vi "Image Processing Module Event Handler.vi"(8 "error in (no error)":errorcluster, 9 "data queue":refnum<queue>, 10 "Data Event":refnum<user-event>) -> ()   [LabVIEW 2018, in "Headless Image Processing Handler.lvclass"]
uses:
  Headless Image Processing Handler.lvclass
  Message/Message.lvclass
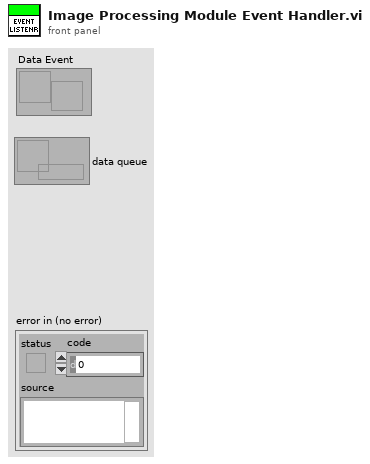
[diagram p1: front panel]
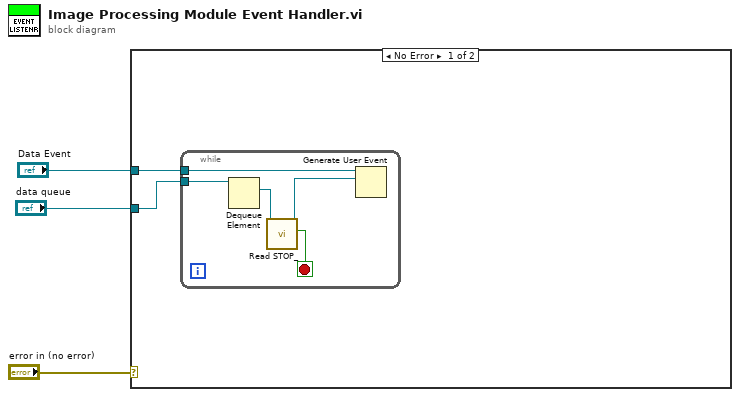
[diagram p0: block diagram]
diagram:
  n1 = case shown="No Error" "error in (no error)" {
    tunnel: "data queue" -> [w4 _]
    tunnel: "Data Event" -> [w5 _]
    frame No Error {
      n2 = while {
        tunnel: w5 -> [w7]
        tunnel: w4 -> [w10]
        stop <- w8 stop-if-true
        n3 = Dequeue Element(queue=w10) -> (element=w9:refnum<class "Message.lvclass">)  [unwired: 2 in, 3 out]
        n4 = call-dynamic "Read STOP_.vi"("Message in"=w9) -> ("STOP?"=w8:bool, "Message out"=w6:refnum<class "Message.lvclass">)  [unwired: 8 in, 1 out]
        n5 = Generate User Event(user event=w7, event data cluster=w6) -> ()  [unwired: 2 in, 2 out]
      }
    }
    frame Error {
    }
  }
